vi "Parse Reponse.vi"(8 "error in":errorcluster, 11 "Input String":string) -> (0 "error out":errorcluster, 1 "Raw Response":string, 3 "Parsed Response":T1)   [LabVIEW 2020, in "driver_flodx_pressure.lvlib"]
uses:
  <instrlib>/RxnRover/FloDx Pressure Driver/driver_flodx_pressure.lvlib
  <instrlib>/RxnRover/FloDx Pressure Driver/Public/Type Defs/ParsedData.ctl
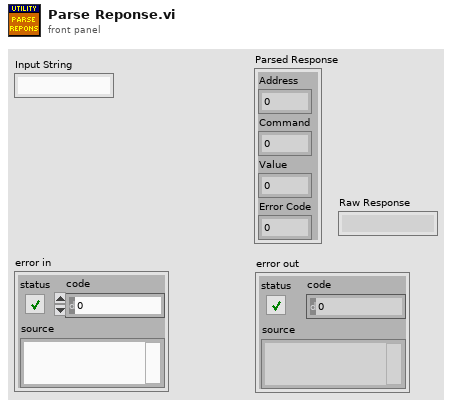
[diagram p1: front panel]
types:
  T1 = cluster{"Address":u32, "Command":u32, "Value":dbl, "Error Code":u32}
  T2 = typedef "driver_flodx_pressure.lvlib/ParsedData.ctl" = cluster{"Address":u32, "Command":u32, "Value":dbl, "Error Code":u32}
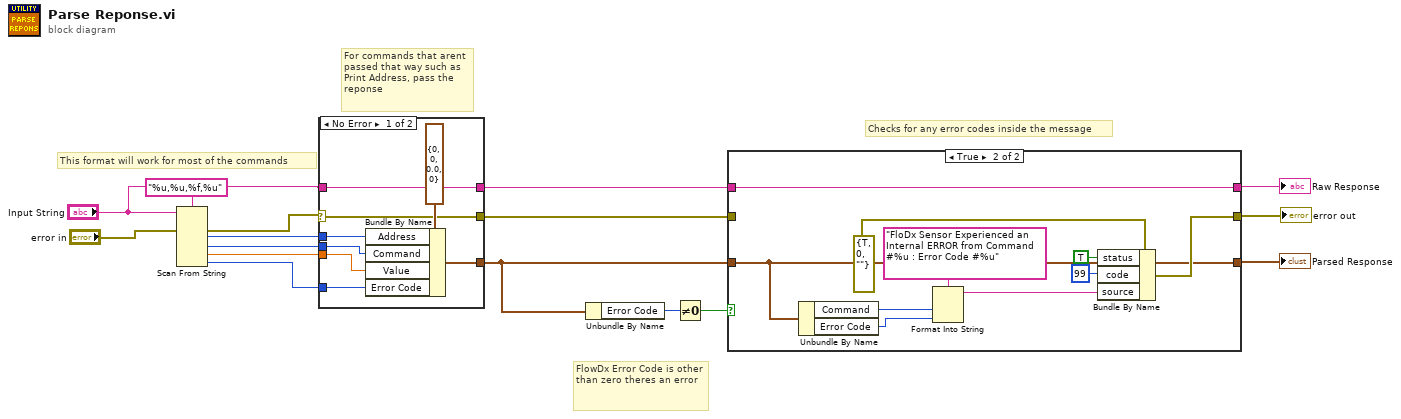
[diagram p0: block diagram]
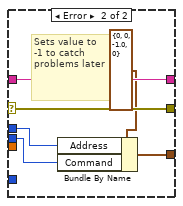
[diagram p3: hidden frame]
diagram:
  # "Checks for any error codes inside the message"
  # "FlowDx Error Code is other than zero theres an error"
  # "For commands that arent passed that way such as Print Address, pass the reponse"
  # "This format will work for most of the commands"
  n1 = Scan From String(format string="%u,%u,%f,%u", input string="Input String", error in="error in") -> (error out=w10:errorcluster, output 1=w15:u32, output 2=w14:u32, output 3=w13:dbl, output 4=w12:u32)  [unwired: 5 in, 2 out]
  n2 = case shown="No Error" w10 {
    selector: w10 -> [w18 w30]
    tunnel: [w24 w28] -> w7
    tunnel: w15 -> [w22 w27]
    tunnel: w14 -> [w21 w26]
    tunnel: w13 -> [w20 _]
    tunnel: w12 -> [w19 _]
    tunnel: [w18 w30] -> w3
    tunnel: [w17 w29] -> w2
    tunnel: "Input String" -> [w17 w29]
    frame No Error {
      n3 = Bundle By Name(cluster=T2 {"Address"=0, "Command"=0, "Value"=0.0, "Error Code"=0} ("Message 2"), "Address"=w22, "Command"=w21, "Value"=w20, "Error Code"=w19) -> (w24:T2)
    }
    frame Error {
      # "Sets value to -1 to catch problems later"
      n4 = Bundle By Name(cluster=T2 {"Address"=0, "Command"=0, "Value"=-1.0, "Error Code"=0} ("Message 2"), "Address"=w27, "Command"=w26) -> (w28:T2)
    }
  }
  n5 = Unbundle By Name(w7) -> ("Error Code"=w1:u32)
  n6 = Not Equal To 0?(x=w1) -> (x != 0?=w8:bool)
  n7 = case shown="True" w8 {
    tunnel: w7 -> [w31 w34]
    tunnel: [w31 w34] -> w6
    tunnel: [w32 w41] -> w5
    tunnel: [w33 w43] -> w4
    tunnel: w3 -> [w32 _]
    tunnel: w2 -> [w33 w43]
    frame False {
    }
    frame True {
      n8 = Unbundle By Name(w34) -> ("Command"=w36:u32, "Error Code"=w35:u32)
      n9 = Format Into String(format string="FloDx Sensor Experienced an Internal ERROR from Command #%u : Error Code #%u", w36, w35) -> (resulting string=w37:string)  [unwired: 2 in, 1 out]
      n10 = Bundle By Name(cluster=errorcluster {"status"=TRUE, "code"=0, "source"=""} ("error IO"), "status"=TRUE, "code"=99, "source"=w37) -> (w41:errorcluster)
    }
  }
  "Parsed Response" <- w6
  "error out" <- w5
  "Raw Response" <- w4
